vi "OpenDevice.vi"() -> (2 "DevIndex":u32, 3 "DevType":u32, 5 "OpenDevice":i32)   [LabVIEW 2016]
uses:
  ECanVci.dll
panel:
  out "Reserved":u32
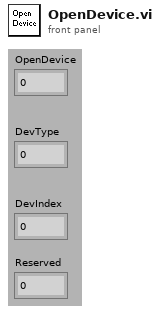
[diagram p1: front panel]
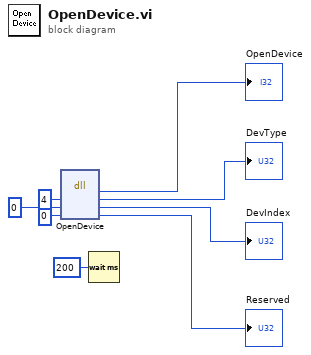
[diagram p0: block diagram]
diagram:
  n1 = dll-call lib="C:/Users/Azmat/Desktop/Labview/ECanVci.dll" fn="OpenDevice"("DevType"=u32 4, "DevIndex"=u32 0, "Reserved"=u32 0) -> ("OpenDevice"=→"OpenDevice":i32, "DevType"=→"DevType":u32, "DevIndex"=→"DevIndex":u32, "Reserved"=→"Reserved":u32)  [unwired: 3 in, 2 out]
  n2 = Wait (ms)(milliseconds to wait=u32 200 ("等待时间（毫秒）")) -> ()  [unwired: 1 out]
